vi "Save To File.vi"(8 "error in (no error)":errorcluster, 11 "Sudoku Class in":refnum<class "Sudoku Class.lvclass">) -> (0 "error out":errorcluster, 3 "Sudoku Class out":refnum<class "Sudoku Class.lvclass">)   [LabVIEW 2015, in "Sudoku Library.lvlib" / "Sudoku Class.lvclass"]
doc: "Created IvanLis by LabVIEW Portal\nProfile: http://labviewportal.org/memberlist.php?mode=viewprofile&u=987\neMail: IvanLisanov@gMail.com\nTelegram: https://t.me/IvanLis"
uses:
  Sudoku Class.lvclass
  Sudoku Class.lvclass/Sudoku Class.ctl
  Sudoku Library.lvlib
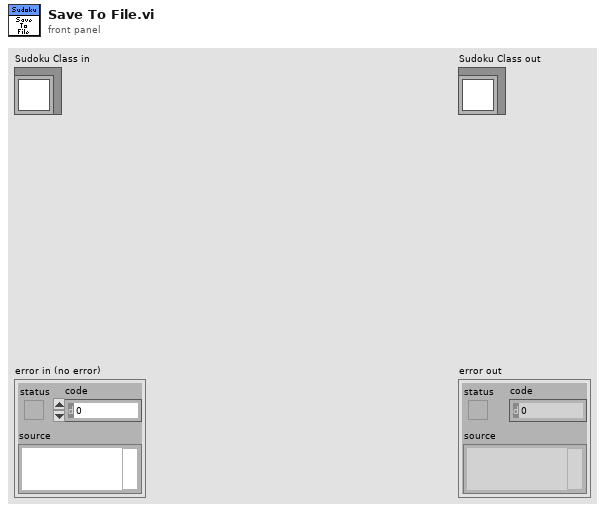
[diagram p1: front panel]
types:
  T1 = typedef "Sudoku Library.lvlib/Sudoku String.ctl" = string[][]
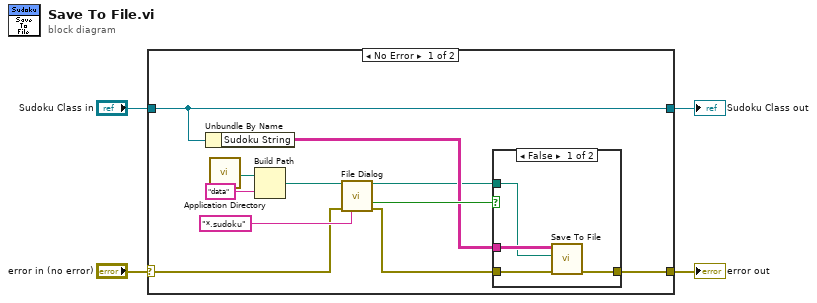
[diagram p0: block diagram]
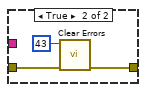
[diagram p2: hidden frame]
diagram:
  n1 = case shown="No Error" "error in (no error)" {
    selector: "error in (no error)" -> [w10 w24]
    tunnel: [w15 w24] -> w3
    tunnel: [w7 w23] -> w1
    tunnel: "Sudoku Class in" -> [w7 w23]
    frame No Error {
      n2 = Unbundle By Name(w7) -> ("Sudoku String"=w6:T1)
      n3 = call <vilib>:"Application Directory.vi"() -> ("Application Directory"=w13:path)
      n4 = Build Path(base path=w13, name or relative path="data") -> (appended path=w11:path)
      n5 = call "File Dialog"("start path"=w11, "error in"=w10, "pattern (all files)"="*.sudoku") -> ("selected path"=w5:path, "cancelled"=w8:bool, "error out"=w9:errorcluster)  [unwired: 9 in, 1 out]
      n6 = case shown="False" w8 {
        tunnel: [w19 w21] -> w15
        tunnel: w9 -> [w18 w22]
        tunnel: w6 -> [w17 _]
        tunnel: w5 -> [w16 _]
        frame False {
          n7 = call "Save To File.vi"("error in (no error)"=w18, "Sudoku File"=w16, "Sudoku String"=w17) -> ("error out"=w19:errorcluster)  [unwired: 8 in]
        }
        frame True {
          n8 = call <vilib>:"Clear Errors.vi"("error in (no error)"=w22, "specific error code to clear (0: all)"=43) -> ("error out"=w21:errorcluster)  [unwired: 4 in, 1 out]
        }
      }
    }
    frame Error {
    }
  }
  "error out" <- w3
  "Sudoku Class out" <- w1
